vi "H5Fget_obj_count.vi"(6 "error in (no error)":errorcluster, 8 "Object types":T1=31 items=["H5F_OBJ_FILE"=1, "H5F_OBJ_DATASET"=2, "H5F_OBJ_GROUP"=4, "H5F_OBJ_DATATYPE"=8, "H5F_OBJ_ATTR"=16, "H5F_OBJ_ALL"=31, "H5F_OBJ_LOCAL"=32], 9 "HDF5 File Ref (All open files)":T2) -> (0 "error out":errorcluster, 2 "Count":i32, 3 "HDF5 Ref out":T2)   [LabVIEW 2017]
doc: "Returns the number of open object identifiers for an open file."
uses:
  <vilib>/UPVI/lvhdf5/library.llb/HDF5 Ref.ctl
  <vilib>/UPVI/lvhdf5/file.llb/H5F_obj_types_t.ctl
  <vilib>/UPVI/lvhdf5/hdf5.dll
panel:
  # "LVHDF5 Toolkit\nCopyright (c) 2005-2013 by Jason D. Sommerville\nCopyright (c) 2014 by UPVI, LLC.\n\nThis use and distribution of this file is governed by the terms found in \nLICENSE.txt distributed with this toolkit and installed at\n <user.lib>\\_lvhdf5\\LICENSE.txt"
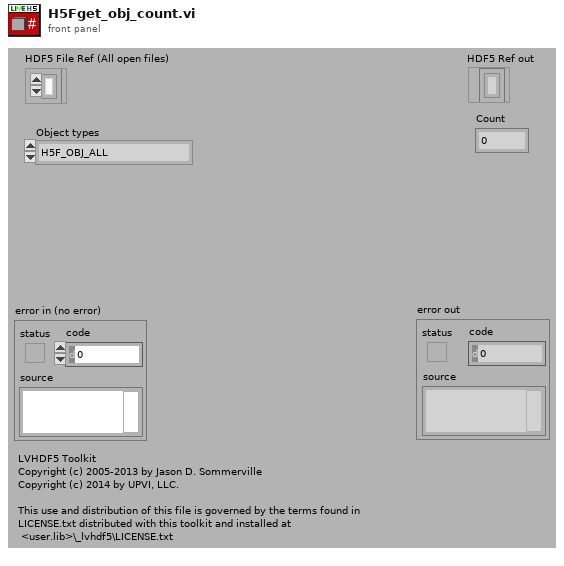
[diagram p1: front panel]
types:
  T1 = typedef "H5F_obj_types_t.ctl" = u32
  T2 = typedef "HDF5 Ref.ctl" = refnum<k1>
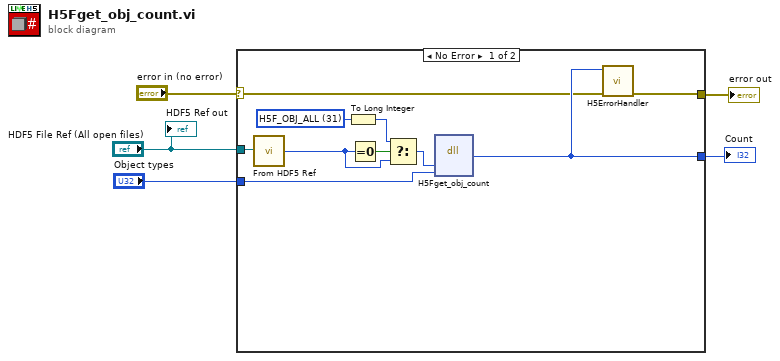
[diagram p0: block diagram]
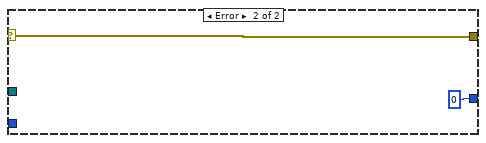
[diagram p2: hidden frame]
diagram:
  n1 = case shown="No Error" "error in (no error)" {
    selector: "error in (no error)" -> [w12 w17]
    tunnel: [w14 w17] -> w4
    tunnel: [w13 0 ("U32")] -> w3
    tunnel: "HDF5 File Ref (All open files)" -> [w15 _]
    tunnel: "Object types" -> [w11 _]
    frame No Error {
      w9 = T1 31 items=["H5F_OBJ_FILE"=1, "H5F_OBJ_DATASET"=2, "H5F_OBJ_GROUP"=4, "H5F_OBJ_DATATYPE"=8, "H5F_OBJ_ATTR"=16, "H5F_OBJ_ALL"=31, "H5F_OBJ_LOCAL"=32] ("Object types")
      n2 = call <vilib>:"From HDF5 Ref.vi"("HDF5 Ref"=w15) -> ("I32"=w8:i32)
      n3 = To Long Integer(number=w9) -> (32bit integer=w10:i32)
      n4 = Equal To 0?(x=w8) -> (x = 0?=w7:bool)
      n5 = Select(t=w10, s=w7, f=w8) -> (s? t:f=w6:i32)
      n6 = dll-call lib="C:/Program Files/National Instruments/LabVIEW 2017/vi.lib/UPVI/lvhdf5/hdf5.dll" fn="H5Fget_obj_count"("file_id"=w6, "types"=w11) -> ("return type"=w13:i64)  [unwired: 5 in, 2 out]
      n7 = call <vilib>:"H5ErrorHandler.vi"("error in (no error)"=w12, "herr_t"=w13) -> ("error out"=w14:errorcluster)  [unwired: 3 in, 4 out]
    }
    frame Error {
    }
  }
  "error out" <- w4
  "Count" <- w3
  "HDF5 Ref out" <- "HDF5 File Ref (All open files)"
